vi "LHF.DB.Mongo.Bson.Variant.vi"(0 "Variant":variant, 5 "error IO":errorcluster) -> (14 "BsonValue":refnum<k24>, 19 "error IO 2":errorcluster)   [LabVIEW 2013, in "LHF.DB.Mongo.lvclass"]
uses:
  LHF.DB.Mongo.lvclass
  C:/Users/schim/Desktop/Projetos/LabVIEW-MongoDB/src/Driver/MongoDB.Bson.dll
  Driver/MongoDB.Bson.dll
  <vilib>/Utility/VariantDataType/VariantType.lvlib
panel:
  in  "Treatment of Infinity/NaN":T1(ring)
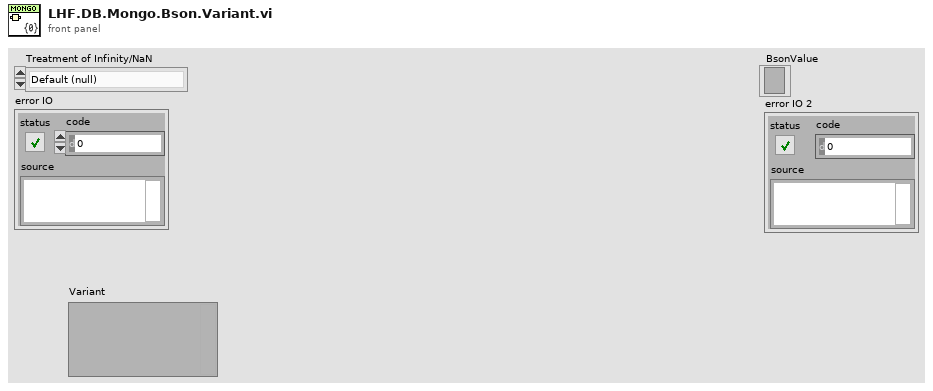
[diagram p1: front panel]
types:
  T1 = enum16{"Default (null)", "Extended", "LabVIEW extensions"}
  T2 = typedef "VariantType.lvlib/Type.ctl" = enum8{"Invalid Type", "Void", "I8", "I16", "I32", "I64", "U8", "U16", "U32", "U64", "Single Float", "Double Float", "Extended Float", "Single Complex", "Double Complex", "Extended Complex", "Enum U8", "Enum U16", "Enum U32", "Enum U64", "Single Float With Unit", "Double Float With Unit", "Extended Float With Unit", "Single Complex with Unit", "Double Complex with Unit", "Extended Complex with Unit", "Boolean", "String", "Path", "Picture", "Tag", "Array", "Cluster", "Variant", "LV Variant", "Waveform", "Timestamp", "Digital Waveform", "Digital Data", "ExpressData", "Refnum", "External Data", "VI", "Poly VI", "LabVIEW Class Instance", "Fixed Point"}
  T3 = typedef "LHF.DB.Mongo.lvclass/LHF.DB.Mongo.Typedef.VariantData.ctl" = cluster{"Type Enum":T2, "Name":string, "Variant":variant}
  T4 = typedef "VariantType.lvlib/RefnumType.ctl" = enum16{"NotARefnum", "UnknownRefnum", "Generic", "Datalog", "ByteStream", "Device", "Occurence", "TCPNetConnection", "Auto", "Menu", "Imaq", "Hardware", "DataSocket", "Visa", "IVI", "UDPNetConnection", "Notifier", "Queue", "Irda", "EventReg", "DotNet", "UserEvent", "Callback", "UNUSED_EMPTY_POSITION", "BlueToothNetConnection", "LVObjApp", "LVObjVI", "LVObjUnknown", "GenericClass", "UserDefinedRefnumTag", "DataValue", "RT FIFO", "TDMS File"}
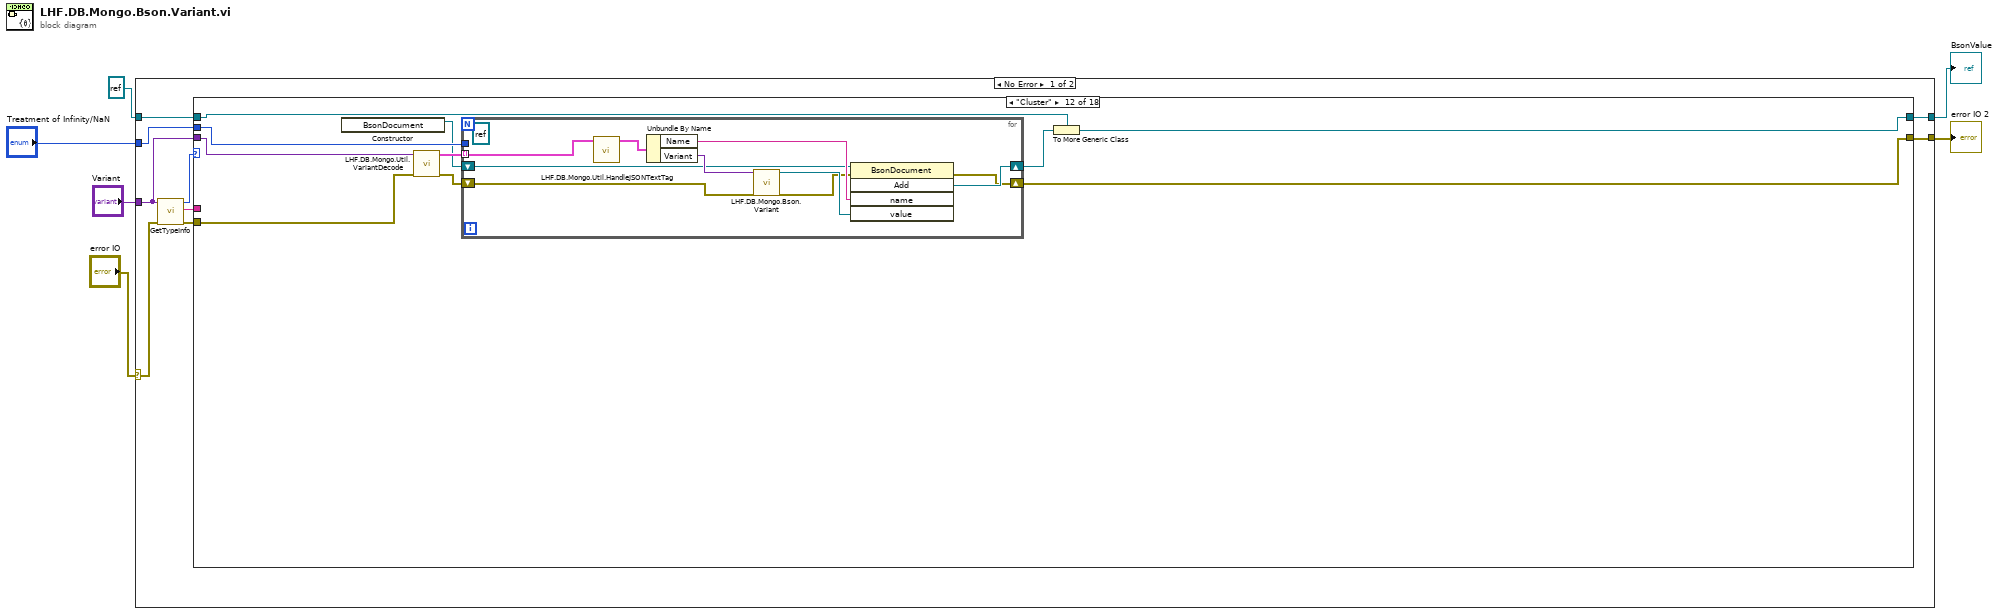
[diagram p0: block diagram]
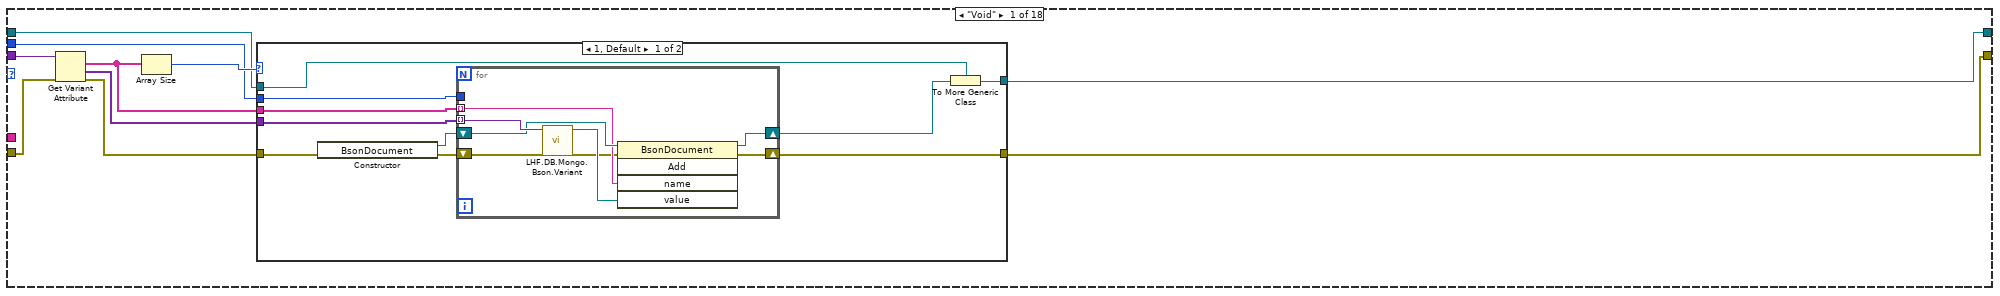
[diagram p2: hidden frame]
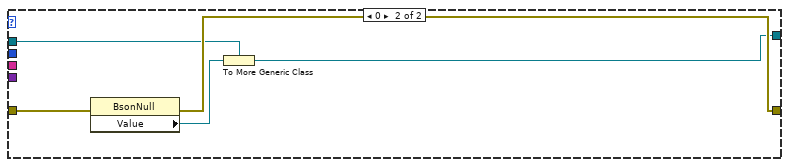
[diagram p3: hidden frame]
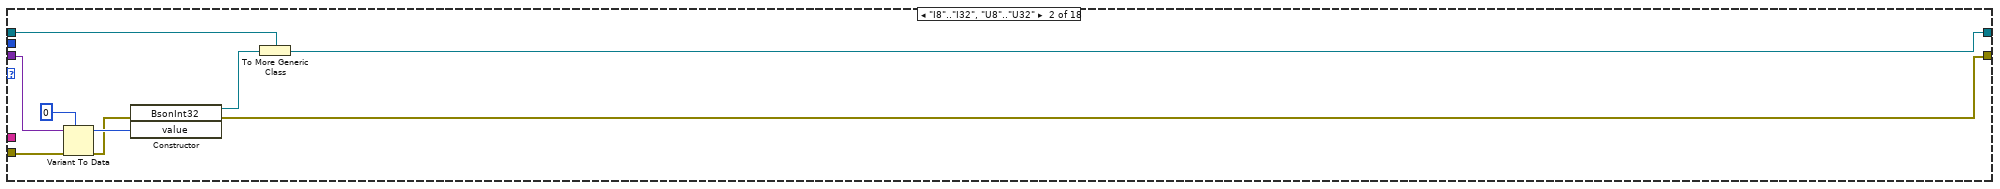
[diagram p4: hidden frame]
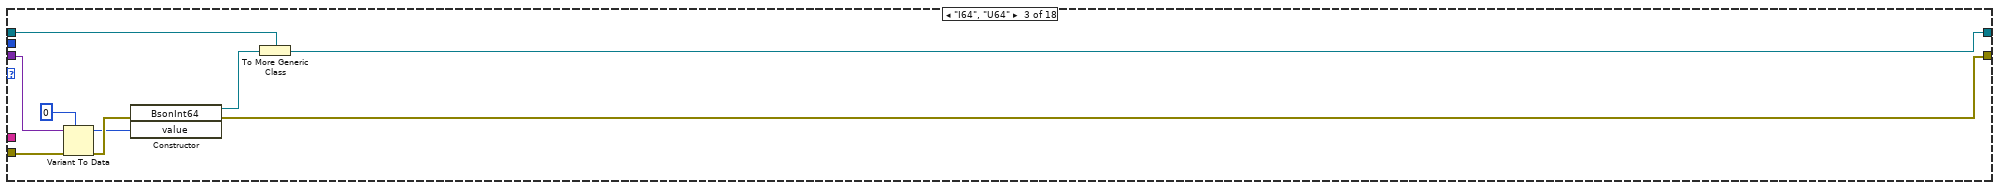
[diagram p5: hidden frame]
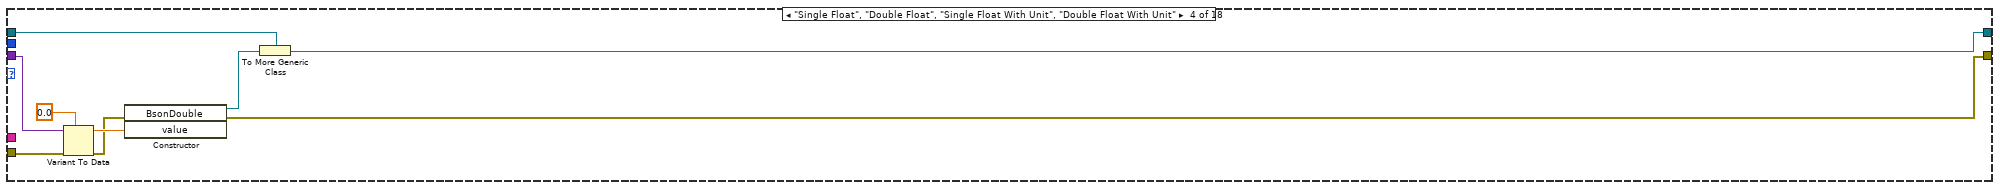
[diagram p6: hidden frame]
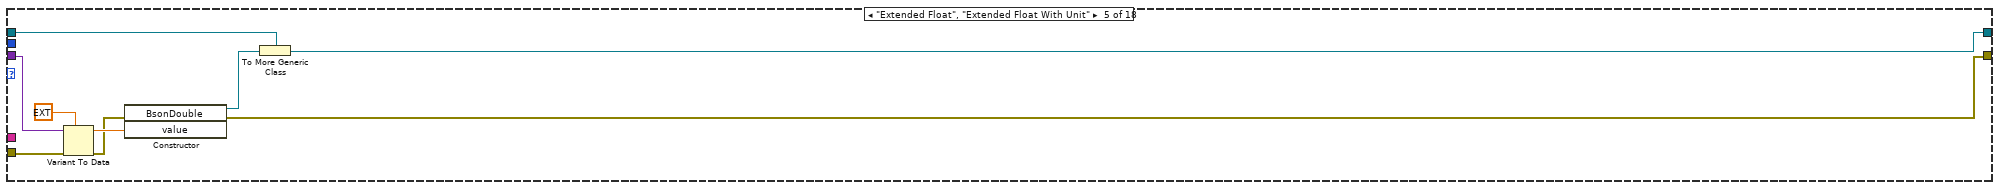
[diagram p7: hidden frame]
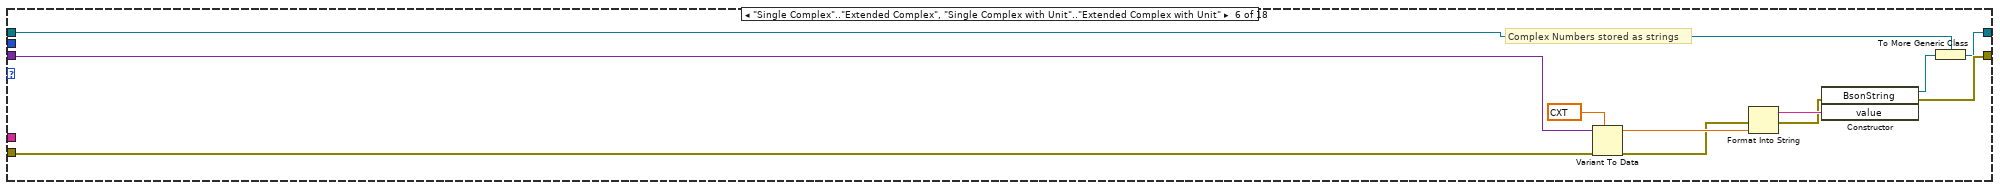
[diagram p8: hidden frame]
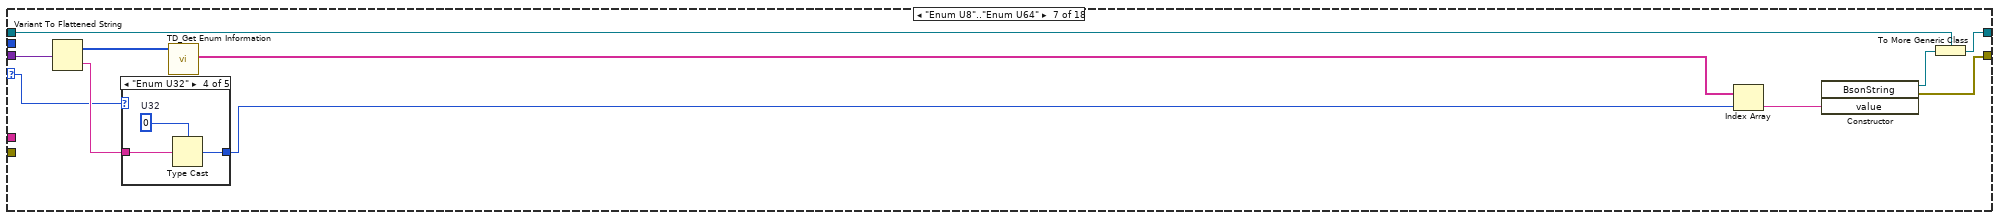
[diagram p9: hidden frame]
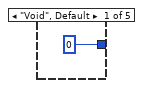
[diagram p10: hidden frame]
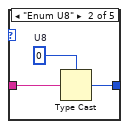
[diagram p11: hidden frame]
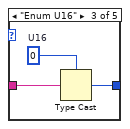
[diagram p12: hidden frame]
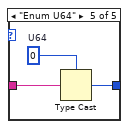
[diagram p13: hidden frame]
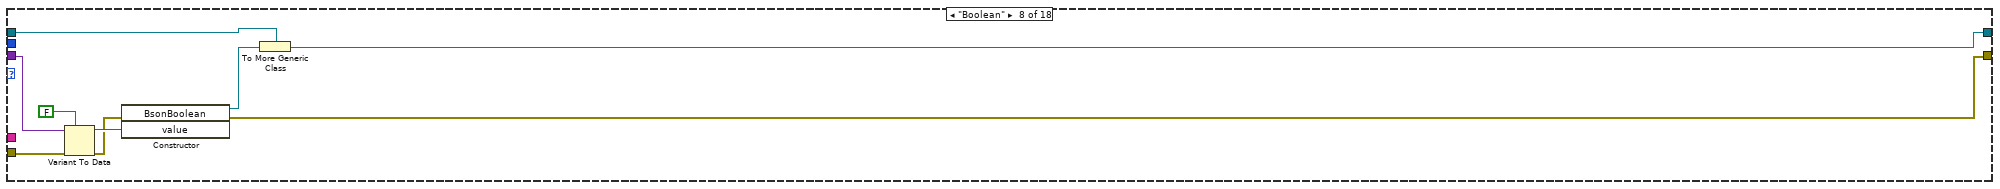
[diagram p14: hidden frame]
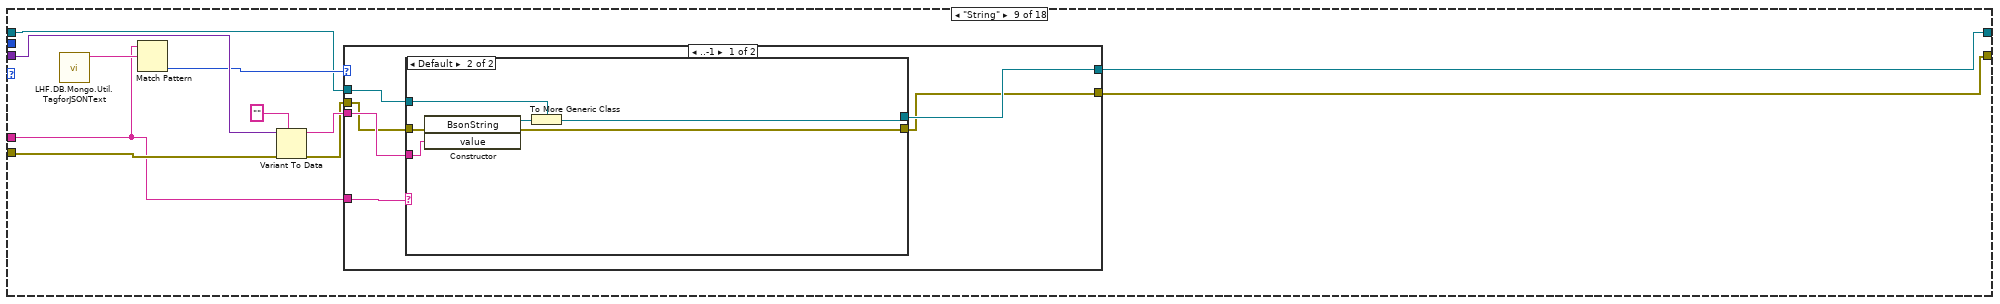
[diagram p15: hidden frame]
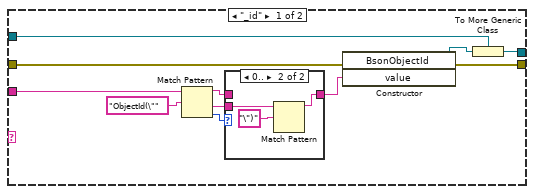
[diagram p16: hidden frame]
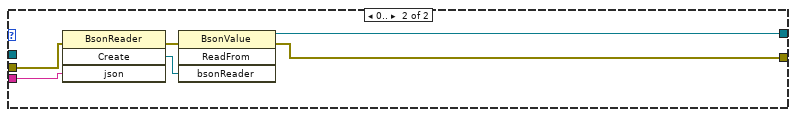
[diagram p18: hidden frame]
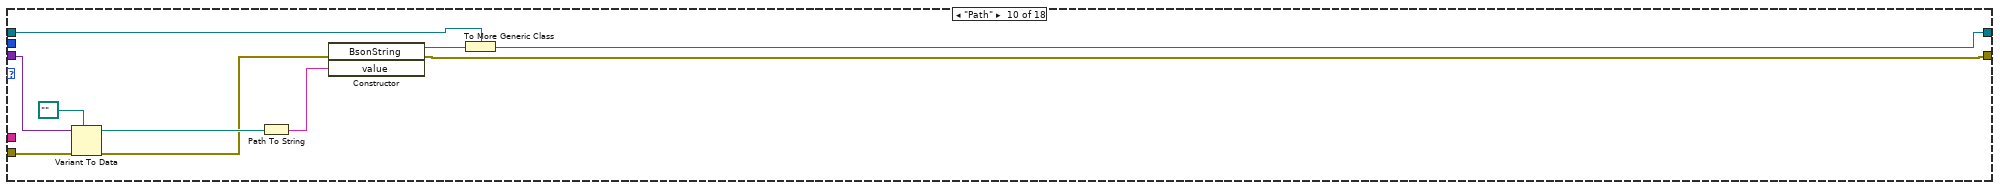
[diagram p19: hidden frame]
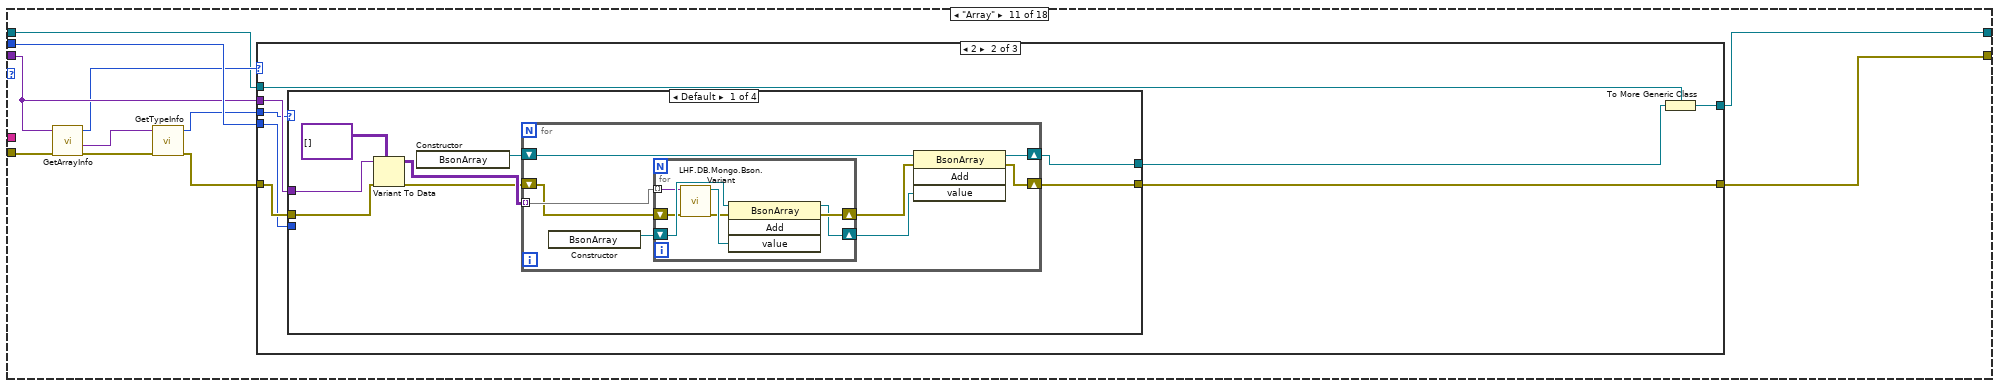
[diagram p20: hidden frame]
diagram:
  n1 = case shown="No Error" "error IO" {
    selector: "error IO" -> [w13 w512]
    tunnel: [w15 w512] -> w1
    tunnel: "Variant" -> [w14 _]
    tunnel: "Treatment of Infinity/NaN" -> [w9 _]
    tunnel: [w8 w511] -> w3
    tunnel: refnum<k24> refnum ("new reference") -> [w7 w511]
    frame No Error {
      n2 = call <vilib>:"GetTypeInfo.vi"("error in (no error)"=w13, "Variant"=w14) -> ("error out"=w12:errorcluster, "Name"=w10:string, "Type Enum"=w11:T2)  [unwired: 5 in, 2 out]
      n3 = case shown="\"Cluster\"" w11 {
        selector: w11 -> [_ _ _ _ _ _ w101 _ _ _ _ _ _ _ _ _ _ _]
        tunnel: w14 -> [w24 w57 w66 w75 w84 w95 w102 w128 w139 w182 w191 w427 w447 w457 w466 w474 w503 w510]
        tunnel: [w25 w52 w63 w68 w79 w88 w98 w122 w135 w176 w193 w429 w443 w452 w461 w468 w495 w506] -> w15
        tunnel: w12 -> [w19 w55 w64 w73 w82 w94 _ w126 w134 w180 w190 w425 w446 w456 w464 w473 w502 w507]
        tunnel: w10 -> [_ _ _ _ _ _ _ _ w129 _ _ _ _ _ _ _ _ _]
        tunnel: w9 -> [w18 _ _ _ _ _ _ _ _ _ w192 w424 _ _ _ _ _ _]
        tunnel: [w16 w49 w58 w67 w76 w85 w96 w120 w131 w173 w183 w420 w440 w449 w459 w467 w493 w504] -> w8
        tunnel: w7 -> [w17 w50 w59 w70 w77 w86 w97 w123 w132 w174 w184 w421 w442 w451 w458 w470 w494 w505]
        frame "Void" {
          n4 = Get Variant Attribute(Variant=w24, error in=w19) -> (names=w22:string[], values=w21:variant[], error out=w20:errorcluster)  [unwired: 2 in, 1 out]
          n5 = Array Size(array=w22) -> (size(s)=w23:i32)
          n6 = case shown="1, Default" w23 {
            tunnel: [w33 w48] -> w25
            tunnel: w22 -> [w34 _]
            tunnel: w21 -> [w35 _]
            tunnel: w20 -> [w26 w47]
            tunnel: w18 -> [w32 _]
            tunnel: w17 -> [w28 w45]
            tunnel: [w29 w44] -> w16
            frame 1, Default {
              n7 = constructor class="BsonDocument"(error in=w26) -> (reference out=w31:refnum<k24>, error out=w27:errorcluster)  [unwired: 2 in, 1 out]
              n8 = for {
                tunnel: w35 -> [w43] mode=indexing
                shift-right: [w36] -> w33
                shift-left: w27 -> [w37]
                tunnel: w34 -> [w40] mode=indexing
                shift-right: [w41] -> w30
                shift-left: w31 -> [w42]
                tunnel: w32 -> [_]
                n9 = call "LHF.DB.Mongo.Bson.Variant.vi"("Variant"=w43, "error IO"=w37) -> ("BsonValue"=w39:refnum<k24>, "error IO 2"=w38:errorcluster)  [unwired: 16 in]
                n10 = invoke class="BsonDocument" method="Add"(reference=w42, error in=w38, "name"=w40, "value"=w39) -> (reference out=w41:refnum<k24>, error out=w36:errorcluster)  [unwired: 1 in, 3 out]
              }
              n11 = To More Generic Class(target class=w28, reference=w30) -> (generic class reference=w29:refnum<k24>)
            }
            frame 0 {
              n12 = property class="BsonNull"(error in=w47) -> (error out=w48:errorcluster, "Value"=w46:refnum<k24>)  [unwired: 1 in, 1 out]
              n13 = To More Generic Class(target class=w45, reference=w46) -> (generic class reference=w44:refnum<k24>)
            }
          }
        }
        frame "I8".."I32", "U8".."U32" {
          n14 = Variant To Data(error in=w55, type=0, Variant=w57) -> (data=w54:i32, error out=w53:errorcluster)
          n15 = constructor class="BsonInt32"(error in=w53, "value"=w54) -> (reference out=w51:refnum<k24>, error out=w52:errorcluster)  [unwired: 2 in, 2 out]
          n16 = To More Generic Class(target class=w50, reference=w51) -> (generic class reference=w49:refnum<k24>)
        }
        frame "I64", "U64" {
          n17 = Variant To Data(error in=w64, type=i64 0, Variant=w66) -> (data=w61:i64, error out=w62:errorcluster)
          n18 = constructor class="BsonInt64"(error in=w62, "value"=w61) -> (reference out=w60:refnum<k24>, error out=w63:errorcluster)  [unwired: 2 in, 2 out]
          n19 = To More Generic Class(target class=w59, reference=w60) -> (generic class reference=w58:refnum<k24>)
        }
        frame "Single Float", "Double Float", "Single Float With Unit", "Double Float With Unit" {
          n20 = Variant To Data(error in=w73, type=sgl 0.0, Variant=w75) -> (data=w72:sgl, error out=w69:errorcluster)
          n21 = constructor class="BsonDouble"(error in=w69, "value"=w72) -> (reference out=w71:refnum<k24>, error out=w68:errorcluster)  [unwired: 2 in, 2 out]
          n22 = To More Generic Class(target class=w70, reference=w71) -> (generic class reference=w67:refnum<k24>)
        }
        frame "Extended Float", "Extended Float With Unit" {
          n23 = Variant To Data(error in=w82, type=ext 0.0, Variant=w84) -> (data=w81:ext, error out=w80:errorcluster)
          n24 = constructor class="BsonDouble"(error in=w80, "value"=w81) -> (reference out=w78:refnum<k24>, error out=w79:errorcluster)  [unwired: 2 in, 2 out]
          n25 = To More Generic Class(target class=w77, reference=w78) -> (generic class reference=w76:refnum<k24>)
        }
        frame "Single Complex".."Extended Complex", "Single Complex with Unit".."Extended Complex with Unit" {
          # "Complex Numbers stored as strings"
          n26 = Variant To Data(error in=w94, type=cxt 0.0+0.0i, Variant=w95) -> (data=w92:cxt, error out=w91:errorcluster)
          n27 = Format Into String(error in=w91, w92) -> (resulting string=w90:string, error out=w89:errorcluster)  [unwired: 2 in]
          n28 = constructor class="BsonString"(error in=w89, "value"=w90) -> (reference out=w87:refnum<k24>, error out=w88:errorcluster)  [unwired: 2 in, 2 out]
          n29 = To More Generic Class(target class=w86, reference=w87) -> (generic class reference=w85:refnum<k24>)
        }
        frame "Enum U8".."Enum U64" {
          n30 = Variant To Flattened String(Variant=w102) -> (data string=w105:string, 1:w106:i16[])
          n31 = case shown="\"Enum U32\"" w101 {
            tunnel: w105 -> [_ w110 w113 w116 w119]
            tunnel: [u64 0 ("U8") w108 w111 w114 w117] -> w103
            frame "Void", Default {
            }
            frame "Enum U8" {
              w109 = u8 0  # U8
              n32 = Type Cast(type=w109, x=w110) -> (*(type *) &x=w108:u8)
            }
            frame "Enum U16" {
              w112 = u16 0  # U16
              n33 = Type Cast(type=w112, x=w113) -> (*(type *) &x=w111:u16)
            }
            frame "Enum U32" {
              w115 = u32 0  # U32
              n34 = Type Cast(type=w115, x=w116) -> (*(type *) &x=w114:u32)
            }
            frame "Enum U64" {
              w118 = u64 0  # U64
              n35 = Type Cast(type=w118, x=w119) -> (*(type *) &x=w117:u64)
            }
          }
          n36 = call <vilib>:"TD_Get Enum Information.vi"("Type descriptor"=w106) -> ("Value Names"=w104:string[])  [unwired: 9 in, 1 out]
          n37 = Index Array(array=w104, index=w103) -> (element=w99:string)
          n38 = constructor class="BsonString"("value"=w99) -> (reference out=w100:refnum<k24>, error out=w98:errorcluster)  [unwired: 3 in, 2 out]
          n39 = To More Generic Class(target class=w97, reference=w100) -> (generic class reference=w96:refnum<k24>)
        }
        frame "Boolean" {
          n40 = Variant To Data(error in=w126, type=FALSE, Variant=w128) -> (data=w124:bool, error out=w121:errorcluster)
          n41 = constructor class="BsonBoolean"(error in=w121, "value"=w124) -> (reference out=w125:refnum<k24>, error out=w122:errorcluster)  [unwired: 2 in, 2 out]
          n42 = To More Generic Class(target class=w123, reference=w125) -> (generic class reference=w120:refnum<k24>)
        }
        frame "String" {
          n43 = call "LHF.DB.Mongo.Util.TagforJSONText.vi"() -> ("Tag for JSON text"=w130:string)  [unwired: 11 in]
          n44 = Match Pattern(string=w129, regular expression=w130) -> (offset past match=w133:i32)  [unwired: 1 in, 3 out]
          n45 = Variant To Data(error in=w134, type="", Variant=w139) -> (data=w137:string, error out=w136:errorcluster)
          n46 = case shown="..-1" w133 {
            tunnel: w137 -> [w145 w172]
            tunnel: w136 -> [w141 w169]
            tunnel: [w142 w168] -> w135
            tunnel: [w144 w167] -> w131
            tunnel: w132 -> [w143 _]
            tunnel: w129 -> [w140 _]
            frame ..-1 {
              n47 = case shown="Default" w140 {
                tunnel: w145 -> [w151 w165]
                tunnel: [w147 w161] -> w144
                tunnel: w143 -> [w146 w164]
                tunnel: [w156 w163] -> w142
                tunnel: w141 -> [w149 w162]
                frame "_id" {
                  n48 = Match Pattern(string=w151, regular expression="ObjectId(\"") -> (before substring=w152:string, after substring=w154:string, offset past match=w153:i32)  [unwired: 1 in, 1 out]
                  n49 = case shown="0.." w153 {
                    tunnel: [w157 w159] -> w150
                    tunnel: w154 -> [_ w158]
                    tunnel: w152 -> [w157 _]
                    frame Default {
                    }
                    frame 0.. {
                      n50 = Match Pattern(string=w158, regular expression="\")") -> (before substring=w159:string)  [unwired: 1 in, 3 out]
                    }
                  }
                  n51 = constructor class="BsonObjectId"(error in=w149, "value"=w150) -> (reference out=w148:refnum<k24>, error out=w156:errorcluster)  [unwired: 2 in, 2 out]
                  n52 = To More Generic Class(target class=w146, reference=w148) -> (generic class reference=w147:refnum<k24>)
                }
                frame Default {
                  n53 = constructor class="BsonString"(error in=w162, "value"=w165) -> (reference out=w166:refnum<k24>, error out=w163:errorcluster)  [unwired: 2 in, 2 out]
                  n54 = To More Generic Class(target class=w164, reference=w166) -> (generic class reference=w161:refnum<k24>)
                }
              }
            }
            frame 0.. {
              n55 = invoke class="BsonReader" method="Create"(error in=w169, "json"=w172) -> (error out=w170:errorcluster, "Create"=w171:refnum<k24>)  [unwired: 2 in, 2 out]
              n56 = invoke class="BsonValue" method="ReadFrom"(error in=w170, "bsonReader"=w171) -> (reference out=w167:refnum<k24>, error out=w168:errorcluster)  [unwired: 2 in, 2 out]
            }
          }
        }
        frame "Path" {
          n57 = Variant To Data(error in=w180, type=path "", Variant=w182) -> (data=w179:path, error out=w177:errorcluster)
          n58 = Path To String(path=w179) -> (string=w178:string)
          n59 = constructor class="BsonString"(error in=w177, "value"=w178) -> (reference out=w175:refnum<k24>, error out=w176:errorcluster)  [unwired: 2 in, 2 out]
          n60 = To More Generic Class(target class=w174, reference=w175) -> (generic class reference=w173:refnum<k24>)
        }
        frame "Array" {
          n61 = call <vilib>:"GetArrayInfo.vi"("error in (no error)"=w190, "Variant"=w191) -> ("error out"=w188:errorcluster, "ArrayElement"=w187:variant, "NDims"=w189:i32)  [unwired: 6 in, 1 out]
          n62 = call <vilib>:"GetTypeInfo.vi"("error in (no error)"=w188, "Variant"=w187) -> ("error out"=w186:errorcluster, "Type Enum"=w185:T2)  [unwired: 5 in, 3 out]
          n63 = case shown="2" w189 {
            tunnel: [w202 w317 w419] -> w193
            tunnel: w192 -> [w201 w315 _]
            tunnel: w191 -> [w203 w318 w415]
            tunnel: w186 -> [w199 w316 w414]
            tunnel: w185 -> [w200 w314 _]
            tunnel: w184 -> [w195 w311 w411]
            tunnel: [w194 w312 w412] -> w183
            frame 1 {
              n64 = constructor class="BsonArray"(error in=w199) -> (reference out=w197:refnum<k24>, error out=w198:errorcluster)  [unwired: 2 in, 1 out]
              n65 = case shown="\"I8\"..\"I32\", \"U8\"..\"U32\"" w200 {
                tunnel: w203 -> [w212 w227 w242 w257 w272 w287 w303]
                tunnel: [w204 w223 w235 w250 w266 w282 w295] -> w202
                tunnel: w198 -> [w208 w225 w240 w255 w270 w283 w299]
                tunnel: w201 -> [w207 _ _ _ _ _ w298]
                tunnel: w197 -> [w206 w221 w238 w254 w268 w281 w297]
                tunnel: [w205 w222 w236 w251 w267 w280 w296] -> w196
                frame Default {
                  n66 = Variant To Data(error in=w208, type=variant[] [], Variant=w212) -> (data=w210:variant[], error out=w209:errorcluster)
                  n67 = for {
                    tunnel: w210 -> [w219] mode=indexing
                    shift-right: [w214] -> w204
                    shift-left: w209 -> [w218]
                    tunnel: w207 -> [_]
                    shift-right: [w215] -> w205
                    shift-left: w206 -> [w216]
                    n68 = call "LHF.DB.Mongo.Bson.Variant.vi"("Variant"=w219, "error IO"=w218) -> ("BsonValue"=w217:refnum<k24>, "error IO 2"=w213:errorcluster)  [unwired: 16 in]
                    n69 = invoke class="BsonArray" method="Add"(reference=w216, error in=w213, "value"=w217) -> (reference out=w215:refnum<k24>, error out=w214:errorcluster)  [unwired: 1 in, 2 out]
                  }
                }
                frame "String" {
                  n70 = Variant To Data(error in=w225, type=string[] [], Variant=w227) -> (data=w224:string[], error out=w220:errorcluster)
                  n71 = for {
                    shift-right: [w232] -> w222
                    shift-left: w221 -> [w234]
                    tunnel: w224 -> [w229] mode=indexing
                    shift-right: [w231] -> w223
                    shift-left: w220 -> [w228]
                    n72 = constructor class="BsonString"(error in=w228, "value"=w229) -> (reference out=w233:refnum<k24>, error out=w230:errorcluster)  [unwired: 2 in, 2 out]
                    n73 = invoke class="BsonArray" method="Add"(reference=w234, error in=w230, "value"=w233) -> (reference out=w232:refnum<k24>, error out=w231:errorcluster)  [unwired: 1 in, 2 out]
                  }
                }
                frame "Single Float".."Extended Float" {
                  n74 = Variant To Data(error in=w240, type=sgl[] [], Variant=w242) -> (data=w237:sgl[], error out=w239:errorcluster)
                  n75 = for {
                    shift-right: [w247] -> w236
                    shift-left: w238 -> [w249]
                    shift-right: [w246] -> w235
                    shift-left: w239 -> [w245]
                    tunnel: w237 -> [w243] mode=indexing
                    n76 = constructor class="BsonDouble"(error in=w245, "value"=w243) -> (reference out=w248:refnum<k24>, error out=w244:errorcluster)  [unwired: 2 in, 2 out]
                    n77 = invoke class="BsonArray" method="Add"(reference=w249, error in=w244, "value"=w248) -> (reference out=w247:refnum<k24>, error out=w246:errorcluster)  [unwired: 1 in, 2 out]
                  }
                }
                frame "I8".."I32", "U8".."U32" {
                  n78 = Variant To Data(error in=w255, type=i32[] [], Variant=w257) -> (data=w252:i32[], error out=w253:errorcluster)
                  n79 = for {
                    shift-right: [w262] -> w251
                    shift-left: w254 -> [w264]
                    shift-right: [w261] -> w250
                    shift-left: w253 -> [w260]
                    tunnel: w252 -> [w258] mode=indexing
                    n80 = constructor class="BsonInt32"(error in=w260, "value"=w258) -> (reference out=w263:refnum<k24>, error out=w259:errorcluster)  [unwired: 2 in, 2 out]
                    n81 = invoke class="BsonArray" method="Add"(reference=w264, error in=w259, "value"=w263) -> (reference out=w262:refnum<k24>, error out=w261:errorcluster)  [unwired: 1 in, 2 out]
                  }
                }
                frame "I64", "U64" {
                  n82 = Variant To Data(error in=w270, type=i64[] [], Variant=w272) -> (data=w265:i64[], error out=w269:errorcluster)
                  n83 = for {
                    shift-right: [w277] -> w267
                    shift-left: w268 -> [w279]
                    shift-right: [w276] -> w266
                    shift-left: w269 -> [w275]
                    tunnel: w265 -> [w273] mode=indexing
                    n84 = constructor class="BsonInt64"(error in=w275, "value"=w273) -> (reference out=w278:refnum<k24>, error out=w274:errorcluster)  [unwired: 2 in, 2 out]
                    n85 = invoke class="BsonArray" method="Add"(reference=w279, error in=w274, "value"=w278) -> (reference out=w277:refnum<k24>, error out=w276:errorcluster)  [unwired: 1 in, 2 out]
                  }
                }
                frame "Timestamp" {
                  n86 = Variant To Data(error in=w283, type=timestamp[] [], Variant=w287) -> (data=w285:timestamp[], error out=w284:errorcluster)
                  n87 = for {
                    tunnel: w285 -> [w294] mode=indexing
                    shift-right: [w288] -> w282
                    shift-left: w284 -> [w293]
                    shift-right: [w290] -> w280
                    shift-left: w281 -> [w291]
                    n88 = call "LHF.DB.Mongo.Bson.Timestamp.vi"("t0"=w294, "error in (no error)"=w293) -> ("BsonString"=w292:refnum<k24>, "error out"=w289:errorcluster)  [unwired: 16 in]
                    n89 = invoke class="BsonArray" method="Add"(reference=w291, error in=w289, "value"=w292) -> (reference out=w290:refnum<k24>, error out=w288:errorcluster)  [unwired: 1 in, 2 out]
                  }
                }
                frame "Waveform" {
                  n90 = Variant To Data(error in=w299, type=waveform(dbl)[] [], Variant=w303) -> (data=w301:waveform(dbl)[], error out=w300:errorcluster)
                  n91 = for {
                    tunnel: w301 -> [w309] mode=indexing
                    shift-right: [w305] -> w295
                    shift-left: w300 -> [w310]
                    tunnel: w298 -> [_]
                    shift-right: [w306] -> w296
                    shift-left: w297 -> [w307]
                    n92 = call "LHF.DB.Mongo.Bson.Waveform.vi"("waveform"=w309, "error in (no error)"=w310) -> ("BsonDocument"=w308:refnum<k24>, "error out"=w304:errorcluster)  [unwired: 16 in]
                    n93 = invoke class="BsonArray" method="Add"(reference=w307, error in=w304, "value"=w308) -> (reference out=w306:refnum<k24>, error out=w305:errorcluster)  [unwired: 1 in, 2 out]
                  }
                }
              }
              n94 = To More Generic Class(target class=w195, reference=w196) -> (generic class reference=w194:refnum<k24>)
            }
            frame 2 {
              n95 = case shown="Default" w314 {
                tunnel: w318 -> [w326 w349 w371 w395]
                tunnel: [w323 w346 w369 w388] -> w317
                tunnel: w316 -> [w325 w348 w372 w391]
                tunnel: w315 -> [_ _ _ _]
                tunnel: [w324 w347 w370 w389] -> w313
                frame Default {
                  n96 = Variant To Data(error in=w325, type=variant[][] [], Variant=w326) -> (data=w322:variant[][], error out=w319:errorcluster)
                  n97 = constructor class="BsonArray"() -> (reference out=w321:refnum<k24>)  [unwired: 3 in, 2 out]
                  n98 = for {
                    tunnel: w322 -> [w334] mode=indexing
                    shift-right: [w331] -> w323
                    shift-left: w319 -> [w327]
                    shift-right: [w328] -> w324
                    shift-left: w321 -> [w329]
                    n99 = constructor class="BsonArray"() -> (reference out=w333:refnum<k24>)  [unwired: 3 in, 2 out]
                    n100 = for {
                      tunnel: w334 -> [w338] mode=indexing
                      shift-right: [w340] -> w332
                      shift-left: w327 -> [w337]
                      shift-right: [w339] -> w330
                      shift-left: w333 -> [w341]
                      n101 = call "LHF.DB.Mongo.Bson.Variant.vi"("Variant"=w338, "error IO"=w337) -> ("BsonValue"=w336:refnum<k24>, "error IO 2"=w335:errorcluster)  [unwired: 16 in]
                      n102 = invoke class="BsonArray" method="Add"(reference=w341, error in=w335, "value"=w336) -> (reference out=w339:refnum<k24>, error out=w340:errorcluster)  [unwired: 1 in, 2 out]
                    }
                    n103 = invoke class="BsonArray" method="Add"(reference=w329, error in=w332, "value"=w330) -> (reference out=w328:refnum<k24>, error out=w331:errorcluster)  [unwired: 1 in, 2 out]
                  }
                }
                frame "Single Float".."Extended Float" {
                  n104 = constructor class="BsonArray"() -> (reference out=w343:refnum<k24>)  [unwired: 3 in, 2 out]
                  n105 = Variant To Data(error in=w348, type=dbl[][] [], Variant=w349) -> (data=w345:dbl[][], error out=w344:errorcluster)
                  n106 = for {
                    tunnel: w345 -> [w357] mode=indexing
                    tunnel: w344 -> [w356]
                    shift-right: [w353] -> w346
                    shift-left: _ -> [_]
                    shift-right: [w350] -> w347
                    shift-left: w343 -> [w351]
                    n107 = constructor class="BsonArray"() -> (reference out=w355:refnum<k24>)  [unwired: 3 in, 2 out]
                    n108 = for {
                      tunnel: w357 -> [w362] mode=indexing
                      shift-right: [w360] -> w354
                      shift-left: w356 -> [w358]
                      shift-right: [w359] -> w352
                      shift-left: w355 -> [w361]
                      n109 = constructor class="BsonDouble"(error in=w358, "value"=w362) -> (reference out=w364:refnum<k24>, error out=w363:errorcluster)  [unwired: 2 in, 2 out]
                      n110 = invoke class="BsonArray" method="Add"(reference=w361, error in=w363, "value"=w364) -> (reference out=w359:refnum<k24>, error out=w360:errorcluster)  [unwired: 1 in, 2 out]
                    }
                    n111 = invoke class="BsonArray" method="Add"(reference=w351, error in=w354, "value"=w352) -> (reference out=w350:refnum<k24>, error out=w353:errorcluster)  [unwired: 1 in, 2 out]
                  }
                }
                frame "I8".."I32", "U8".."U32" {
                  n112 = Variant To Data(error in=w372, type=i32[][] [], Variant=w371) -> (data=w368:i32[][], error out=w367:errorcluster)
                  n113 = constructor class="BsonArray"() -> (reference out=w366:refnum<k24>)  [unwired: 3 in, 2 out]
                  n114 = for {
                    tunnel: w368 -> [w380] mode=indexing
                    tunnel: w367 -> [w379]
                    shift-right: [w376] -> w369
                    shift-left: _ -> [_]
                    shift-right: [w373] -> w370
                    shift-left: w366 -> [w374]
                    n115 = constructor class="BsonArray"() -> (reference out=w378:refnum<k24>)  [unwired: 3 in, 2 out]
                    n116 = for {
                      tunnel: w380 -> [w385] mode=indexing
                      shift-right: [w383] -> w377
                      shift-left: w379 -> [w381]
                      shift-right: [w382] -> w375
                      shift-left: w378 -> [w384]
                      n117 = constructor class="BsonInt32"(error in=w381, "value"=w385) -> (reference out=w387:refnum<k24>, error out=w386:errorcluster)  [unwired: 2 in, 2 out]
                      n118 = invoke class="BsonArray" method="Add"(reference=w384, error in=w386, "value"=w387) -> (reference out=w382:refnum<k24>, error out=w383:errorcluster)  [unwired: 1 in, 2 out]
                    }
                    n119 = invoke class="BsonArray" method="Add"(reference=w374, error in=w377, "value"=w375) -> (reference out=w373:refnum<k24>, error out=w376:errorcluster)  [unwired: 1 in, 2 out]
                  }
                }
                frame "I64", "U64" {
                  n120 = Variant To Data(error in=w391, type=i64[][] [], Variant=w395) -> (data=w393:i64[][], error out=w392:errorcluster)
                  n121 = constructor class="BsonArray"() -> (reference out=w390:refnum<k24>)  [unwired: 3 in, 2 out]
                  n122 = for {
                    tunnel: w393 -> [w403] mode=indexing
                    tunnel: w392 -> [w402]
                    shift-right: [w399] -> w388
                    shift-left: _ -> [_]
                    shift-right: [w396] -> w389
                    shift-left: w390 -> [w397]
                    n123 = constructor class="BsonArray"() -> (reference out=w401:refnum<k24>)  [unwired: 3 in, 2 out]
                    n124 = for {
                      tunnel: w403 -> [w408] mode=indexing
                      shift-right: [w406] -> w400
                      shift-left: w402 -> [w404]
                      shift-right: [w405] -> w398
                      shift-left: w401 -> [w407]
                      n125 = constructor class="BsonInt64"(error in=w404, "value"=w408) -> (reference out=w410:refnum<k24>, error out=w409:errorcluster)  [unwired: 2 in, 2 out]
                      n126 = invoke class="BsonArray" method="Add"(reference=w407, error in=w409, "value"=w410) -> (reference out=w405:refnum<k24>, error out=w406:errorcluster)  [unwired: 1 in, 2 out]
                    }
                    n127 = invoke class="BsonArray" method="Add"(reference=w397, error in=w400, "value"=w398) -> (reference out=w396:refnum<k24>, error out=w399:errorcluster)  [unwired: 1 in, 2 out]
                  }
                }
              }
              n128 = To More Generic Class(target class=w311, reference=w313) -> (generic class reference=w312:refnum<k24>)
            }
            frame Default {
              n129 = call "LHF.DB.Mongo.Util.VariantDecode.vi"("error in (no error)"=w414, "variant"=w415) -> ("error out"=w418:errorcluster, "Array Dimensions (Reversed)"=w416:i32[], "Variant Data"=w417:T3[])  [unwired: 7 in]
              n130 = call "LHF.DB.Mongo.Bson.MultiDArray.vi"("error in (no error)"=w418, "Array Dimensions"=w416, "Variant Data"=w417) -> ("error out"=w419:errorcluster, "BsonArray"=w413:refnum<k24>)  [unwired: 6 in, 1 out]
              n131 = To More Generic Class(target class=w411, reference=w413) -> (generic class reference=w412:refnum<k24>)
            }
          }
        }
        frame "Cluster" {
          (unwired) refnum<k24> refnum ("new reference")
          n132 = constructor class="BsonDocument"() -> (reference out=w423:refnum<k24>)  [unwired: 3 in, 2 out]
          n133 = call "LHF.DB.Mongo.Util.VariantDecode.vi"("error in (no error)"=w425, "variant"=w427) -> ("error out"=w426:errorcluster, "Variant Data"=w428:T3[])  [unwired: 7 in, 1 out]
          n134 = for {
            shift-right: [w433] -> w422
            shift-left: w423 -> [w432]
            shift-right: [w431] -> w429
            shift-left: w426 -> [w434]
            tunnel: w428 -> [w439] mode=indexing
            tunnel: w424 -> [_]
            n135 = call "LHF.DB.Mongo.Util.HandleJSONTextTag.vi"("Variant Data"=w439) -> ("Variant Data (tag stripped)"=w438:T3)  [unwired: 9 in, 1 out]
            n136 = Unbundle By Name(w438) -> ("Name"=w437:string, "Variant"=w436:variant)
            n137 = call "LHF.DB.Mongo.Bson.Variant.vi"("Variant"=w436, "error IO"=w434) -> ("BsonValue"=w435:refnum<k24>, "error IO 2"=w430:errorcluster)  [unwired: 16 in]
            n138 = invoke class="BsonDocument" method="Add"(reference=w432, error in=w430, "name"=w437, "value"=w435) -> (error out=w431:errorcluster, "Add"=w433:refnum<k24>)  [unwired: 1 in, 3 out]
          }
          n139 = To More Generic Class(target class=w421, reference=w422) -> (generic class reference=w420:refnum<k24>)
        }
        frame "Variant", "LV Variant" {
          n140 = Variant To Data(error in=w446, type=variant, Variant=w447) -> (data=w445:variant, error out=w444:errorcluster)
          n141 = call "LHF.DB.Mongo.Bson.Variant.vi"("Variant"=w445, "error IO"=w444) -> ("BsonValue"=w441:refnum<k24>, "error IO 2"=w443:errorcluster)  [unwired: 16 in]
          n142 = To More Generic Class(target class=w442, reference=w441) -> (generic class reference=w440:refnum<k24>)
        }
        frame "Waveform" {
          n143 = Variant To Data(error in=w456, type=waveform(dbl) {"t0"=timestamp(0 s since 1904-01-01), "dt"=1.0, "Y"=[]} ("waveform"), Variant=w457) -> (data=w454:waveform(dbl), error out=w450:errorcluster)
          n144 = call "LHF.DB.Mongo.Bson.Waveform.vi"("waveform"=w454, "error in (no error)"=w450) -> ("BsonDocument"=w453:refnum<k24>, "error out"=w452:errorcluster)  [unwired: 16 in]
          n145 = To More Generic Class(target class=w451, reference=w453) -> (generic class reference=w449:refnum<k24>)
        }
        frame "Timestamp" {
          n146 = Variant To Data(error in=w464, type=timestamp(0 s since 1904-01-01), Variant=w466) -> (data=w463:timestamp, error out=w462:errorcluster)
          n147 = call "LHF.DB.Mongo.Bson.Timestamp.vi"("t0"=w463, "error in (no error)"=w462) -> ("BsonString"=w460:refnum<k24>, "error out"=w461:errorcluster)  [unwired: 16 in]
          n148 = To More Generic Class(target class=w458, reference=w460) -> (generic class reference=w459:refnum<k24>)
        }
        frame "Refnum" {
          n149 = call <vilib>:"GetRefnumInfo.vi"("error in (no error)"=w473, "Variant"=w474) -> ("error out"=w476:errorcluster, "ReferenceType"=w475:T4)  [unwired: 6 in, 2 out]
          n150 = case shown="Default" w475 {
            selector: w475 -> [w479 _ _]
            tunnel: [w478 w482 w486] -> w471
            tunnel: w476 -> [w480 w484 w488]
            tunnel: [w477 w481 w487] -> w469
            tunnel: w474 -> [_ w485 w491]
            frame "NotARefnum", "UnknownRefnum" {
              n151 = call <userlib>:"Get Strings from Enum__ogtk.vi"("error in (no error)"=w480, "Enum"=w479) -> ("error out"=w477:errorcluster, "String Value"=w478:string)  [unwired: 6 in, 2 out]
            }
            frame "Visa", "IVI", "UserDefinedRefnumTag" {
              n152 = Variant To Data(error in=w484, type="", Variant=w485) -> (data=w482:string, error out=w481:errorcluster)
            }
            frame Default {
              n153 = Variant To Flattened String(Variant=w491) -> (data string=w490:string)  [unwired: 1 out]
              n154 = Type Cast(type=0, x=w490) -> (*(type *) &x=w489:i32)
              n155 = Format Into String(error in=w488, w489) -> (resulting string=w486:string, error out=w487:errorcluster)  [unwired: 2 in]
            }
          }
          n156 = constructor class="BsonString"(error in=w469, "value"=w471) -> (reference out=w472:refnum<k24>, error out=w468:errorcluster)  [unwired: 2 in, 2 out]
          n157 = To More Generic Class(target class=w470, reference=w472) -> (generic class reference=w467:refnum<k24>)
        }
        frame "LabVIEW Class Instance" {
          n158 = Variant To Data(error in=w502, type=refnum<class> refnum ("LabVIEW Object"), Variant=w503) -> (data=w500:refnum<class>, error out=w496:errorcluster)
          n159 = Flatten To String(anything=w500, error in (no error)=w496) -> (data string=w498:string, error out=w497:errorcluster)  [unwired: 2 in, 1 out]
          n160 = constructor class="BsonString"(error in=w497, "value"=w498) -> (reference out=w499:refnum<k24>, error out=w495:errorcluster)  [unwired: 2 in, 2 out]
          n161 = To More Generic Class(target class=w494, reference=w499) -> (generic class reference=w493:refnum<k24>)
        }
        frame Default {
          n162 = Variant To Flattened String(Variant=w510) -> (data string=w508:string)  [unwired: 1 out]
          n163 = constructor class="BsonString"(error in=w507, "value"=w508) -> (reference out=w509:refnum<k24>, error out=w506:errorcluster)  [unwired: 2 in, 2 out]
          n164 = To More Generic Class(target class=w505, reference=w509) -> (generic class reference=w504:refnum<k24>)
        }
      }
    }
    frame Error {
    }
  }
  "BsonValue" <- w3
  "error IO 2" <- w1
